vi "AB_Source_Delete_Property.vi"(8 "error in (no error)":errorcluster, 10 "type":T2, 11 "sourceProperties in":T1[](array[typedef])) -> (0 "error out":errorcluster, 1 "deletedProperty":T1={"sourcePropertyType"=enum."Password", "value"=variant}, 2 "found":bool, 3 "sourceProperties out":T1[](array[typedef]))   [LabVIEW 2020]
uses:
  <vilib>/AppBuilder/AB_Source_Properties.ctl
  <vilib>/AppBuilder/AB_Source_Property_Type.ctl
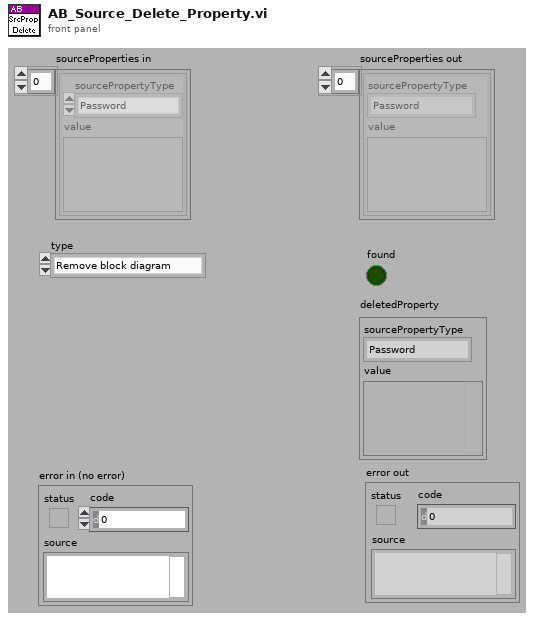
[diagram p1: front panel]
types:
  T1 = typedef "AB_Source_Properties.ctl" = cluster{"sourcePropertyType":T2, "value":variant}
  T2 = typedef "AB_Source_Property_Type.ctl" = enum16{"Remove block diagram", "Remove front panel", "Password", "Window has title bar", "Show menu bar", "Show vertical scroll bar", "Show horizontal scroll bar", "Show toolbar", "Show Abort button", "Show fp when called", "Window behavior", "Allow user to close window", "Window run-time position", "Run when opened", "Allow debugging", "Auto error handling", "Generate guard code", "Use stack variables", "Expression folding", "Integer only", "Inline subVI"}
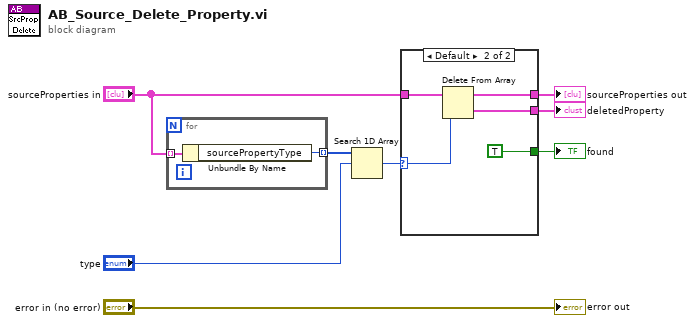
[diagram p0: block diagram]
diagram:
  n1 = for {
    tunnel: "sourceProperties in" -> [w10] mode=indexing
    tunnel: [w9] -> w8 mode=indexing
    n2 = Unbundle By Name(w10) -> ("sourcePropertyType"=w9:T2)
  }
  n3 = Search 1D Array(1D array=w8, element="type") -> (index of element=w6:i32)  [unwired: 1 in]
  n4 = case shown="Default" w6 {
    selector: w6 -> [_ w13]
    tunnel: "sourceProperties in" -> [w11 w15]
    tunnel: [_ TRUE] -> w5
    tunnel: [w11 w14] -> w2
    tunnel: [_ w12] -> w1
    frame -1 {
    }
    frame Default {
      n5 = Delete From Array(array=w15, index=w13) -> (deleted portion=w12:T1, array with subset deleted=w14:T1[])  [unwired: 1 in]
    }
  }
  "sourceProperties out" <- w2
  "found" <- w5
  "deletedProperty" <- w1
  "error out" <- "error in (no error)"
